vi "PFD_AirspeedSpeed.vi"(8 "Refresh Rate (Hz)":u32=60, 10 "Airspeedminmax":cluster{"Max":i16, "Min":i16, "Show":bool}={"Max"=6, "Min"=0, "Show"=TRUE}) -> (3 "Airspeed":picture, 11 "AirSpeed":dbl)   [LabVIEW 2023]
uses:
  PFD_Global.vi
panel:
  in  "stop":bool
  out "AIRSPEED":bool
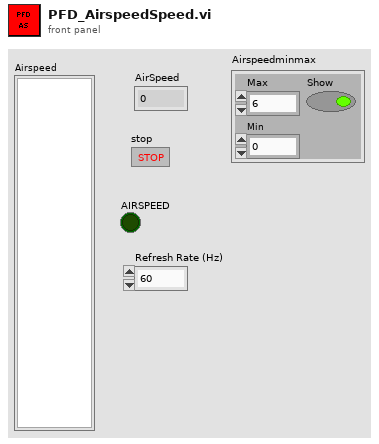
[diagram p1: front panel]
types:
  T1 = cluster{"left":i16, "top":i16, "right":i16, "bottom":i16}
  T2 = cluster{"Width":u16, "Style":enum32{"Solid", "Dash", "Dot", "DashDot", "DashDotDot"}}
  T3 = cluster{"horizontal":enum16{"left", "center", "right"}, "vertical":enum16{"top", "center", "bottom"}}
  T4 = cluster{"Font Name:":string, "Size":i16, "Strikeout?":bool, "Italic?":bool, "Underline?":bool, "Outline?":bool, "Shadow?":bool, "Bold?":bool}
  T5 = enum16{"User-specified Font", "Application Font", "System Font", "Dialog Font"}
  T6 = cluster{cluster{"Width 3":i16, i16}, cluster{"Width 4":i16, i16}}
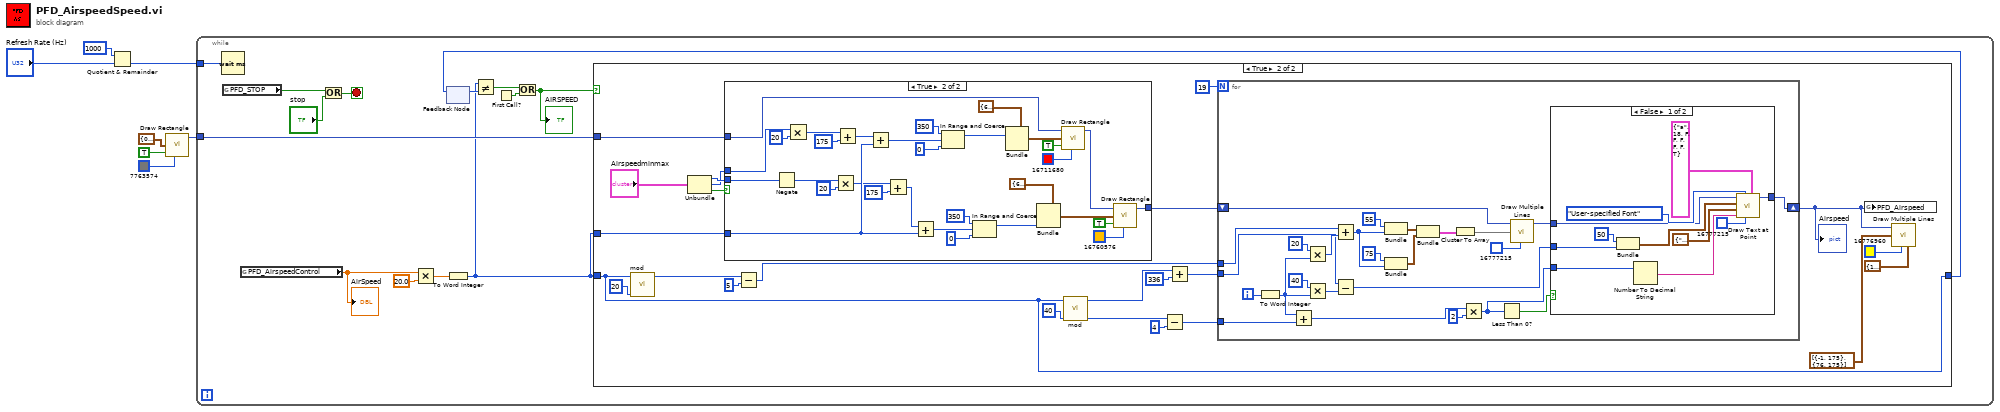
[diagram p0: block diagram]
diagram:
  n1 = Quotient & Remainder(x=u32 1000, y="Refresh Rate (Hz)") -> (floor(x/y)=w1:u32)  [unwired: 1 out]
  n2 = call <vilib>:"Draw Rectangle.vi"("rect"=T1 {"left"=0, "top"=0, "right"=75, "bottom"=350}, "fill?(F)"=TRUE, "color(black)"=u32 7763574 ("Speed_color_background")) -> ("new picture"=w7:picture)  [unwired: 6 in]
  n3 = while {
    tunnel: w7 -> [w17]
    tunnel: w1 -> [w8]
    stop <- w16 stop-if-true
    n4 = Wait (ms)(milliseconds to wait=w8) -> ()  [unwired: 1 out]
    n5 = global read "PFD_Global.vi" "PFD_STOP"() -> (w10:bool)
    n6 = global read "PFD_Global.vi" "PFD_AirspeedControl"() -> (w11:dbl)
    "AirSpeed" <- w11
    n7 = Or(x=w10, y="stop") -> (x .or. y?=w16:bool)
    n8 = Multiply(x=w11, y=20.0) -> (x*y=w12:dbl)
    n9 = feedback #1() -> (w20:i16)  [unwired: 1 in]
    n10 = To Word Integer(number=w12) -> (16bit integer=w13:i16)
    n11 = Not Equal?(x=w13, y=w20) -> (x != y?=w19:bool)
    n12 = First Call?() -> (First Call?: T/F=w18:bool)
    n13 = Or(x=w19, y=w18) -> (x .or. y?=w15:bool)
    "AIRSPEED" <- w15
    n14 = case shown="True" w15 {
      tunnel: w13 -> [w22 w31]
      tunnel: [w22 w31] -> w21
      tunnel: w13 -> [_ w30]
      tunnel: w17 -> [_ w28]
      frame False {
      }
      frame True {
        n15 = call "mod.vi"("Divide"=i16 20 ("x"), "Value In"=w31) -> ("Value out"=w35:i16)  [unwired: 8 in, 1 out]
        n16 = Unbundle("Airspeedminmax") -> ("Max"=w27:i16, "Min"=w26:i16, "Show"=w25:bool)
        n17 = case shown="True" w25 {
          tunnel: w30 -> [_ w76]
          tunnel: w26 -> [_ w72]
          tunnel: w27 -> [_ w67]
          tunnel: [w47 w77] -> w29
          tunnel: w28 -> [w47 w48]
          frame False {
          }
          frame True {
            n18 = Negate(x=w67) -> (-x=w70:i16)
            n19 = Multiply(x=w72, y=i16 20) -> (x*y=w75:i16)
            n20 = Multiply(x=w70, y=i16 20) -> (x*y=w68:i16)
            n21 = Add(x=w75, y=i16 175 ("top")) -> (x+y=w74:i16)
            n22 = Add(x=w74, y=w76) -> (x+y=w54:i16)
            n23 = Add(x=w68, y=i16 175) -> (x+y=w69:i16)
            n24 = Add(x=w69, y=w76) -> (x+y=w50:i16)
            n25 = In Range and Coerce(upper limit=i16 350, x=w54, lower limit=i16 0) -> (coerced(x)=w53:i16)  [unwired: 1 out]
            n26 = In Range and Coerce(upper limit=i16 350, x=w50, lower limit=i16 0) -> (coerced(x)=w49:i16)  [unwired: 1 out]
            n27 = Bundle(cluster=T1 {"left"=60, "top"=175, "right"=76, "bottom"=350} ("rect"), "top"=w53) -> (w61:T1)  [unwired: 3 in]
            n28 = Bundle(cluster=T1 {"left"=60, "top"=0, "right"=76, "bottom"=75} ("rect 2"), "bottom"=w49) -> (w57:T1)  [unwired: 3 in]
            n29 = call <vilib>:"Draw Rectangle.vi"("picture"=w48, "rect"=w61, "fill?(F)"=TRUE, "color(black)"=u32 16711680) -> ("new picture"=w78:picture)  [unwired: 5 in]
            n30 = call <vilib>:"Draw Rectangle.vi"("picture"=w78, "rect"=w57, "fill?(F)"=TRUE, "color(black)"=u32 16760576) -> ("new picture"=w77:picture)  [unwired: 5 in]
          }
        }
        n31 = Subtract(x=w35, y=i16 5) -> (x-y=w32:i16)
        n32 = call "mod.vi"("Divide"=i16 40, "Value In"=w31) -> ("Ceil"=w42:i16, "Value out"=w41:i16)  [unwired: 8 in]
        n33 = Subtract(x=w42, y=i16 4) -> (x-y=w36:i16)
        n34 = Add(x=w41, y=i16 336) -> (x+y=w37:i16)
        n35 = for {
          N: 19 -> [_]
          shift-right: [w85] -> w23
          shift-left: w29 -> [w95]
          tunnel: w37 -> [w87]
          tunnel: w36 -> [w86]
          tunnel: w32 -> [w82]
          i -> [w84]
          n36 = To Word Integer(number=w84) -> (16bit integer=w83:i16)
          n37 = Add(x=w83, y=w86) -> (x+y=w92:i16)
          n38 = Multiply(x=i16 20, y=w83) -> (x*y=w97:i16)
          n39 = Multiply(x=i16 40 ("Divide"), y=w83) -> (x*y=w94:i16)
          n40 = Add(x=w82, y=w97) -> (x+y=w80:i16)
          n41 = Subtract(x=w87, y=w94) -> (x-y=w93:i16)
          n42 = Bundle("Width 3"=i16 55, w80) -> (w102:cluster{"Width 3":i16, i16})  [unwired: 1 in]
          n43 = Bundle("Width 4"=i16 75, w80) -> (w101:cluster{"Width 4":i16, i16})  [unwired: 1 in]
          n44 = Bundle(w102, w101) -> (w103:T6)  [unwired: 1 in]
          n45 = Cluster To Array(cluster=w103) -> (array=w99:cluster{"Width 4":i16, i16}[])
          n46 = Multiply(x=w92, y=i16 2) -> (x*y=w90:i16)
          n47 = Less Than 0?(x=w90) -> (x < 0?=w89:bool)
          n48 = call <vilib>:"Draw Multiple Lines.vi"("picture"=w95, "line endpoints"=w99, "color(black)"=u32 16777215) -> ("new picture"=w79:picture)  [unwired: 6 in]
          n49 = case shown="False" w89 {
            tunnel: w79 -> [w111 w115]
            tunnel: [w110 w115] -> w85
            tunnel: w93 -> [w105 _]
            tunnel: w90 -> [w104 _]
            frame False {
              n50 = Bundle("Width 3"=i16 50, w105) -> (w108:cluster{"Width 3":i16, i16})  [unwired: 1 in]
              n51 = Number To Decimal String(number=w104) -> (decimal integer string=w106:string)  [unwired: 1 in]
              n52 = call <vilib>:"Draw Text at Point.vi"("[user-specified font]"=T4 {"Font Name:"="a", "Size"=18, "Strikeout?"=FALSE, "Italic?"=FALSE, "Underline?"=FALSE, "Outline?"=FALSE, "Shadow?"=FALSE, "Bold?"=TRUE}, "text color(black)"=u32 16777215, "desired font(Application)"=T5."User-specified Font", "text"=w106, "alignment(left, top)"=T3 {"horizontal"=enum."right", "vertical"=enum."center"}, "origin"=w108, "picture"=w111) -> ("new picture"=w110:picture)  [unwired: 3 in, 1 out]
            }
            frame True {
            }
          }
        }
        "Airspeed" <- w23
        n53 = global write "PFD_Global.vi" "PFD_Airspeed"(w23) -> ()
        n54 = call <vilib>:"Draw Multiple Lines.vi"("picture"=w23, "line endpoints"=cluster{"x":i16, "y":i16}[] [{"x"=-1, "y"=175}, {"x"=76, "y"=175}], "color(black)"=u32 16776960, "pen"=T2 {"Width"=1, "Style"=enum."Solid"}) -> ()  [unwired: 5 in, 1 out]
      }
    }
    n55 = feedback-in #1(w21) -> ()
  }
